vi "GetImage.vi"(0 "XRef":T5, 1 "State In":T3) -> (14 "Image":T2, 15 "Fatal Error Out":T1)   [LabVIEW 2018, in "RetryNode.xnode"]
uses:
  RetryNode.xnode
  <vilib>/XNodeSupport/XNodeXNodeRef.ctl
  State.ctl
  <vilib>/Utility/miscctls.llb/LVRectTypeDef.ctl
  <vilib>/XNodeSupport/XNodeImage.ctl
  <vilib>/XNodeSupport/XNodeErrorCluster.ctl
  <vilib>/XNodeSupport/NI_XNodeSupport.lvlib
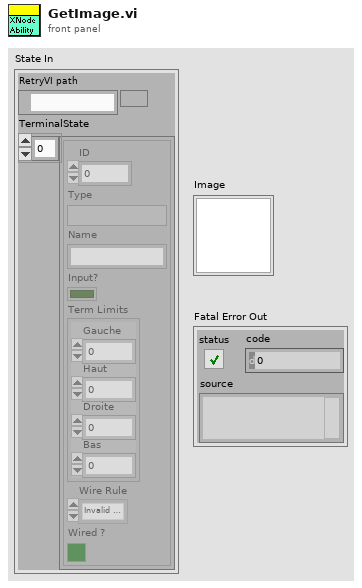
[diagram p1: front panel]
types:
  T1 = typedef "NI_XNodeSupport.lvlib/XNodeErrorCluster.ctl" = errorcluster
  T2 = typedef "NI_XNodeSupport.lvlib/XNodeImage.ctl" = picture
  T3 = typedef "RetryNode.xnode/State.ctl" = cluster{"RetryVI path":path, "TerminalState":cluster{"ID":i32, "Type":variant, "Name":string, "Input?":bool, "Term Limits":T4, "Wire Rule":enum16{"Invalid Wire Rule", "Required", "Recommended", "Optional", "Dynamic Dispatch"}, "Wired ?":bool}[]}
  T4 = typedef "LVRectTypeDef.ctl" = cluster{"Left":i16, "Top":i16, "Right":i16, "Bottom":i16}
  T5 = typedef "NI_XNodeSupport.lvlib/XNodeXNodeRef.ctl" = refnum<vi>
  T6 = cluster{"Width":i16, "Style":enum32{"Solid", "Dash", "Dot", "DashDot", "DashDotDot"}}
  T7 = cluster{"left":i16, "top":i16, "right":i16, "bottom":i16}
  T8 = typedef "imagedata.ctl" = cluster{"image type":i32, "image depth":i32, "image":u8[], "mask":u8[], "colors":u32[], "Rectangle":cluster{"left":i16, "top":i16, "right":i16, "bottom":i16}}
  T9 = cluster{"left":i32, "top":i32, "right":i32, "bottom":i32}
  T10 = typedef "LVBoundsTypeDef.ctl" = cluster{"Width":u32, "Height":u32}
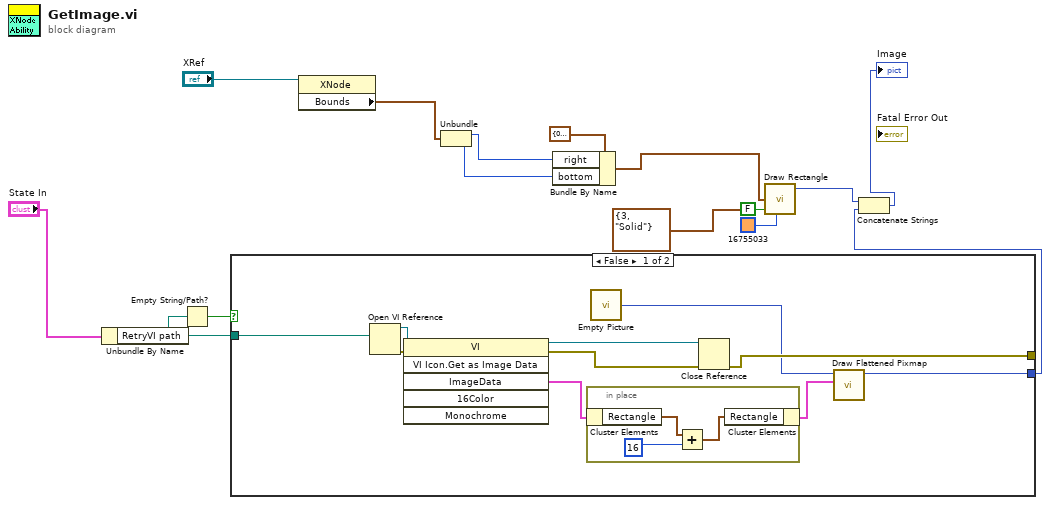
[diagram p0: block diagram]
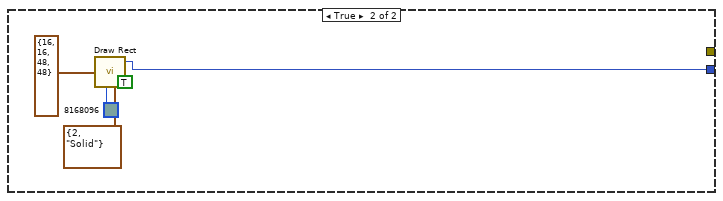
[diagram p2: hidden frame]
diagram:
  n1 = Unbundle By Name("State In") -> ("RetryVI path"=w14:path)
  n2 = Empty String/Path?(string/path=w14) -> (empty?=w15:bool)
  n3 = case shown="False" w15 {
    tunnel: w14 -> [w23 _]
    tunnel: [w22 w29] -> w3
    tunnel: [w19 _] -> _
    frame False {
      n4 = Open VI Reference(vi path=w23) -> (vi reference=w25:refnum<vi>, error out=w24:errorcluster)  [unwired: 5 in]
      n5 = invoke class="VI" method="VI Icon.Get as Image Data"(reference=w25, error in=w24) -> (reference out=w20:refnum<vi>, error out=w21:errorcluster, "ImageData"=w18:T8)  [unwired: 4 in, 3 out]
      n6 = in-place {
        n7 = in-place-cluster #1(w18) -> ("Rectangle"=w28:T7)
        n8 = Add(x=w28, y=16) -> (x+y=w27:T9)
        n9 = in-place-cluster #1("Rectangle"=w27) -> (w17:T8)
      }
      n10 = call "Empty Picture"() -> ("empty picture"=w16:picture)
      n11 = Close Reference(reference=w20, error in (no error)=w21) -> (error out=w19:errorcluster)
      n12 = call <vilib>:"Draw Flattened Pixmap.vi"("image data"=w17, "picture"=w16) -> ("new picture"=w22:picture)  [unwired: 7 in]
    }
    frame True {
      n13 = call <vilib>:"Draw Rect.vi"("rect"=T7 {"left"=16, "top"=16, "right"=48, "bottom"=48}, "fill?(F)"=TRUE, "color(black)"=u32 8168096, "pen"=T6 {"Width"=2, "Style"=enum."Solid"}) -> ("new picture"=w29:picture)  [unwired: 5 in]
    }
  }
  n14 = property class="XNode"(reference="XRef") -> ("Bounds"=w7:T10)  [unwired: 1 in, 2 out]
  n15 = Unbundle(w7) -> ("Width"=w6:u32, "Height"=w5:u32)
  n16 = Bundle By Name(cluster=T7 {"left"=0, "top"=0, "right"=0, "bottom"=0} ("rect"), "right"=w6, "bottom"=w5) -> (w10:T7)
  n17 = call <vilib>:"Draw Rectangle.vi"("rect"=w10, "fill?(F)"=FALSE, "color(black)"=u32 16755033, "pen"=T6 {"Width"=3, "Style"=enum."Solid"}) -> ("new picture"=w4:picture)  [unwired: 5 in]
  n18 = Concatenate Strings(w4, w3) -> (→"Image":picture)
